vi "think_and_act_with_mark_253.vi"(8 "error in (no error)":errorcluster, 9 "antState":T1, 10 "pieceOfWorld":T4[][](array[typedef]), 11 "Igor in":refnum<class "Igor.lvclass">) -> (0 "error out":errorcluster, 2 "action":T2, 3 "Igor out":refnum<class "Igor.lvclass">)   [LabVIEW 2015]
doc: "Ant thinks and chooses action\nCreated by Artem Shevelev\nshevelev.pro\nartem@shevelev.pro\nLabVIEW Portal: https://labviewportal.org/memberlist.php?mode=viewprofile&u=2340"
uses:
  ant_base/ant_base.lvclass
  ant_base/actionType_enum.ctl
  ant_base/action_cluster.ctl
  actors/world/typedefs/markValue.ctl
  actors/world/world.lvlib
  Igor.lvclass
  moving/move_forvard.vi
  moving/move_back.vi
  actors/world/typedefs/amountOfFood.ctl
  actors/world/typedefs/markValue_cluster.ctl
  actors/world/typedefs/anthillType_enum.ctl
  actors/world/typedefs/worldCell_cluster.ctl
  ant_base/antState_cluster.ctl
  actors/world/typedefs/markVolume.ctl
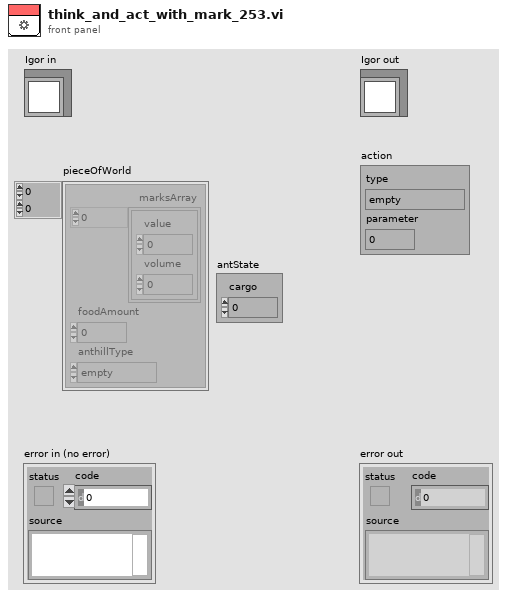
[diagram p1: front panel]
types:
  T1 = typedef "ant_base.lvclass/antState_cluster.ctl" = cluster{"cargo":u8}
  T2 = typedef "ant_base.lvclass/action_cluster.ctl" = cluster{"type":T3, "parameter":dbl}
  T3 = typedef "ant_base.lvclass/actionType_enum.ctl" = enum8{"empty", "move", "take", "put", "mark"}
  T4 = typedef "world.lvlib/worldCell_cluster.ctl" = cluster{"marksArray":T5[], "foodAmount":T8, "anthillType":T9}
  T5 = typedef "world.lvlib/markValue_cluster.ctl" = cluster{"value":T6, "volume":T7}
  T6 = typedef "world.lvlib/markValue.ctl" = u8
  T7 = typedef "world.lvlib/markVolume.ctl" = u16
  T8 = typedef "world.lvlib/amountOfFood.ctl" = i32
  T9 = typedef "world.lvlib/anthillType_enum.ctl" = enum16{"empty", "own", "rival"}
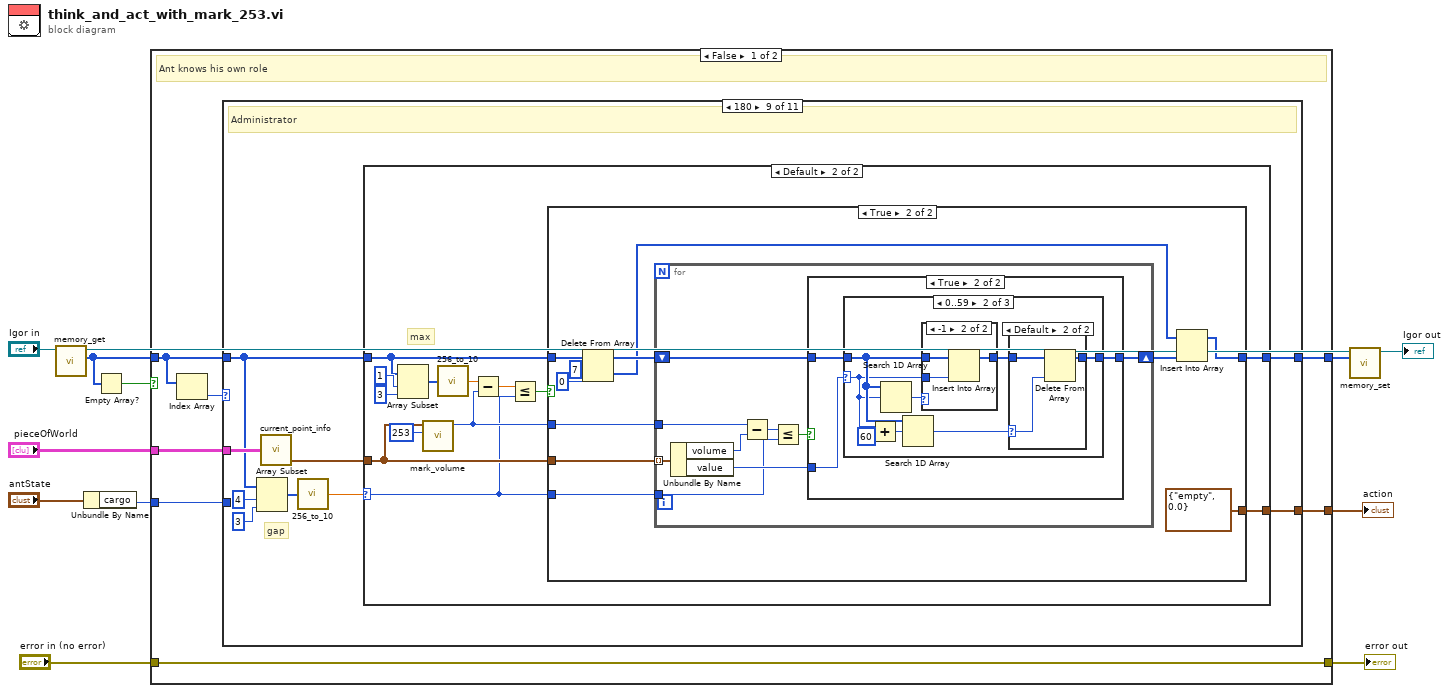
[diagram p0: block diagram]
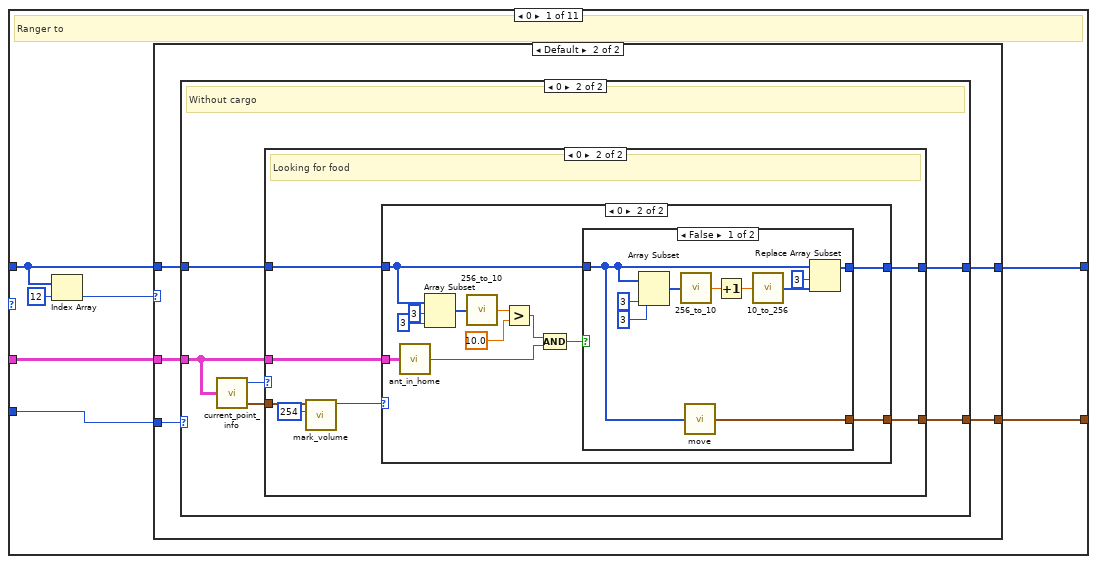
[diagram p2: hidden frame]
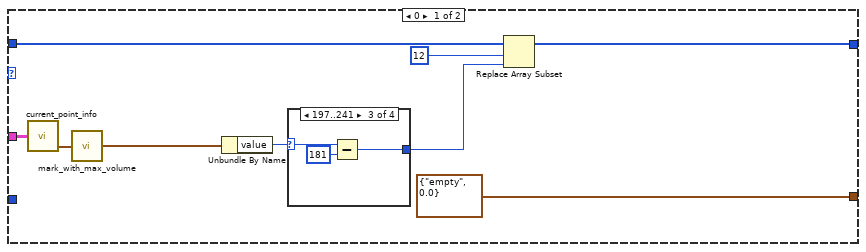
[diagram p3: hidden frame]
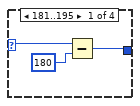
[diagram p4: hidden frame]
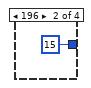
[diagram p5: hidden frame]
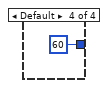
[diagram p6: hidden frame]
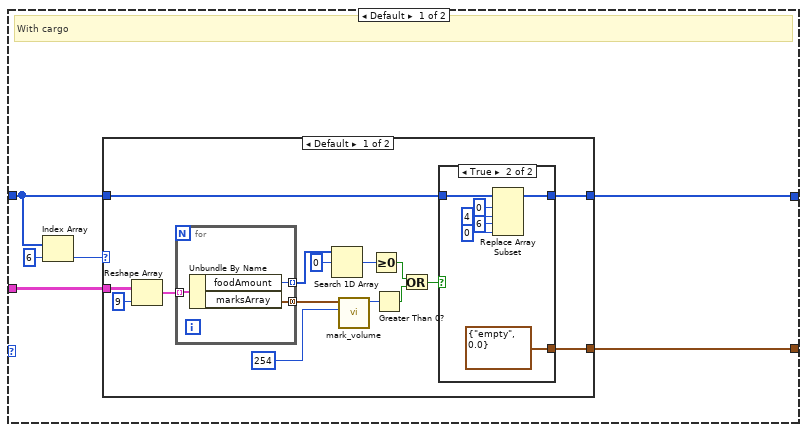
[diagram p7: hidden frame]
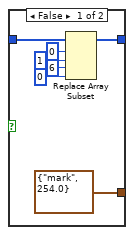
[diagram p8: hidden frame]
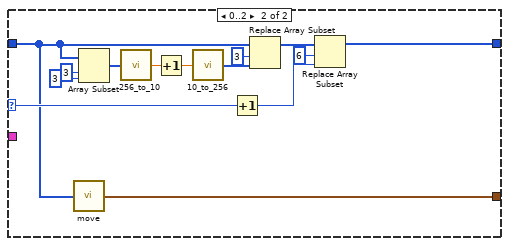
[diagram p9: hidden frame]
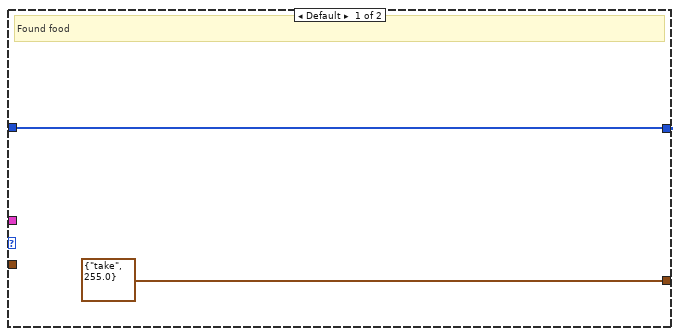
[diagram p10: hidden frame]
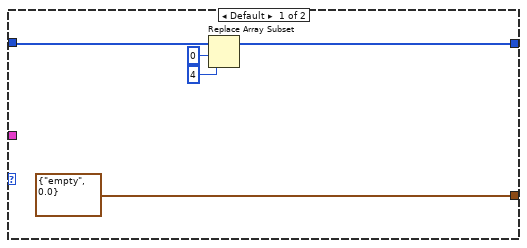
[diagram p11: hidden frame]
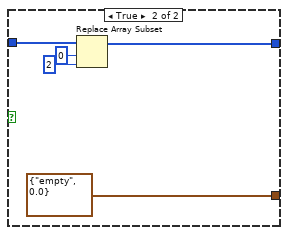
[diagram p12: hidden frame]
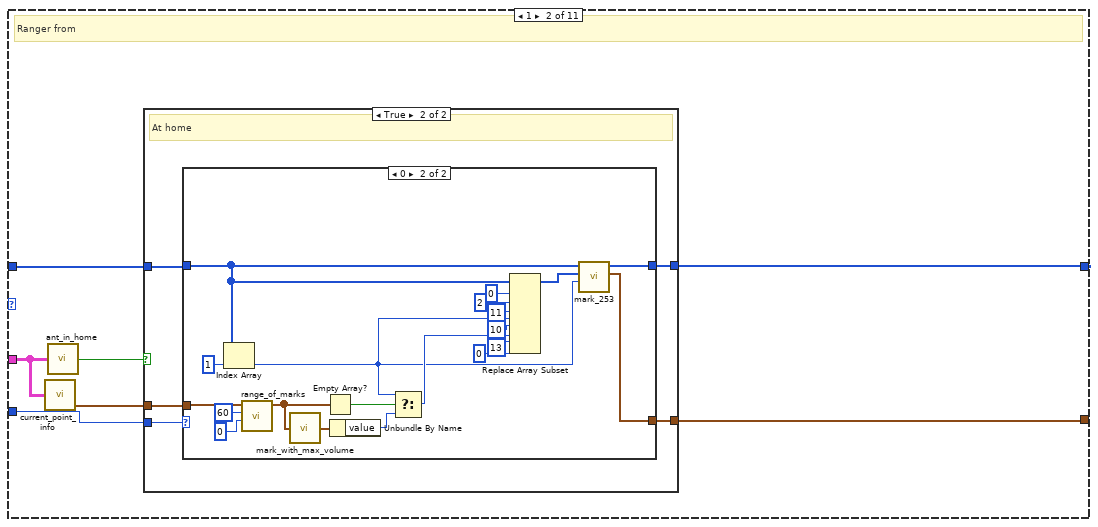
[diagram p13: hidden frame]
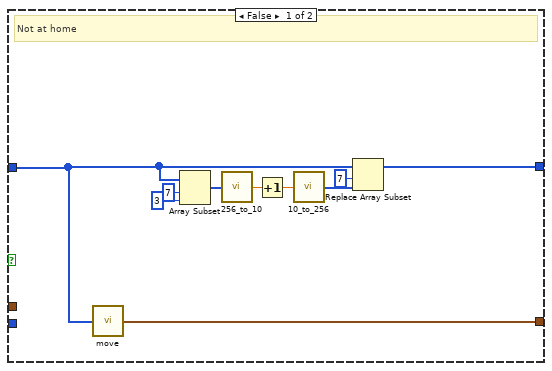
[diagram p14: hidden frame]
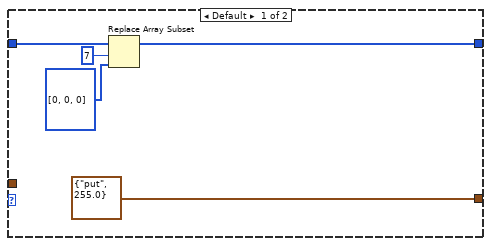
[diagram p15: hidden frame]
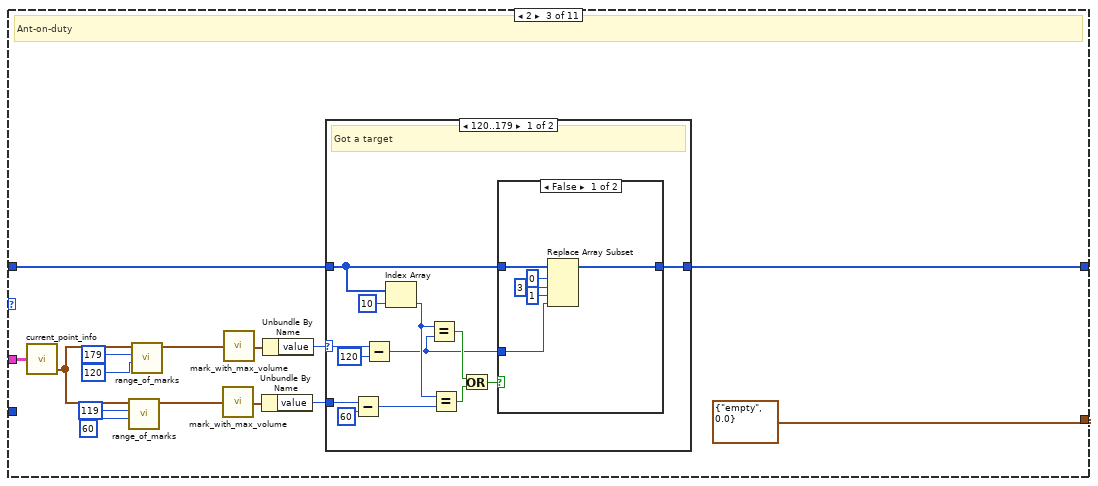
[diagram p16: hidden frame]
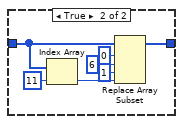
[diagram p17: hidden frame]
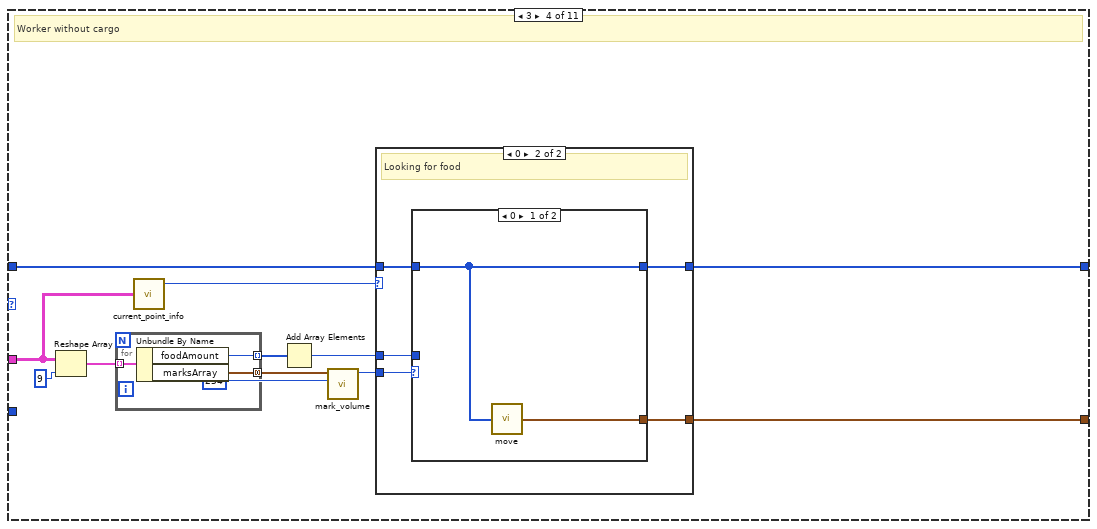
[diagram p19: hidden frame]
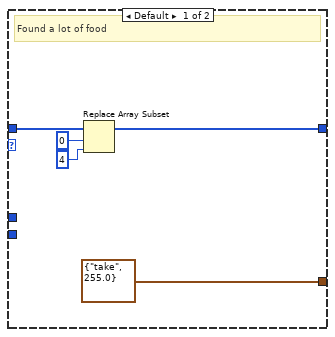
[diagram p20: hidden frame]
diagram:
  n1 = call "memory_get.vi"("ant_base in"="Igor in") -> ("memory"=w2:u8[], "ant_base out"=w7:refnum<class "Igor.lvclass">)  [unwired: 8 in, 1 out]
  n2 = Unbundle By Name("antState") -> ("cargo"=w3:u8)
  n3 = Empty Array?(array=w2) -> (empty?=w9:bool)
  n4 = case shown="False" w9 {
    tunnel: [w19 w757] -> w4
    tunnel: [w17 w756] -> w12
    tunnel: "error in (no error)" -> [w19 w757]
    tunnel: w2 -> [w16 w753]
    tunnel: "pieceOfWorld" -> [w15 w752]
    tunnel: [w14 w754] -> w6
    tunnel: w3 -> [w13 _]
    frame False {
      # "Ant knows his own role"
      n5 = Index Array(array=w16) -> (element=w18:u8)  [unwired: 1 in]
      n6 = case shown="180" w18 {
        tunnel: [w26 w154 T2 {"type"=enum."empty", "parameter"=0.0} ("action") w247 w282 w315 w445 w497 w560 w680 T2 {"type"=enum."empty", "parameter"=0.0} ("action")] -> w17
        tunnel: w16 -> [w22 w148 w207 w248 w281 w314 w448 w498 w556 w676 w749]
        tunnel: w15 -> [w23 w150 w206 w238 w279 w311 w444 w494 w558 w678 _]
        tunnel: [w25 w153 w208 w245 w280 w316 w446 w496 w559 w679 w749] -> w14
        tunnel: w13 -> [w24 w152 _ _ _ _ w449 _ _ _ _]
        frame 0 {
          # "Ranger to"
          n7 = Index Array(array=w22, index=12) -> (element=w20:u8)
          n8 = case shown="Default" w20 {
            tunnel: [T2 {"type"=enum."empty", "parameter"=0.0} ("action") w48] -> w26
            tunnel: w22 -> [w31 w47]
            tunnel: [w30 w46] -> w25
            tunnel: w24 -> [_ w45]
            tunnel: w23 -> [w34 w44]
            frame 0 {
              n9 = call "current_point_info.vi"("pieceOfWorld"=w34) -> ("marksArray"=w33:T5[])  [unwired: 2 out]
              n10 = call "mark_with_max_volume.vi"("marksArray"=w33) -> ("markValue"=w32:T5)
              n11 = Unbundle By Name(w32) -> ("value"=w28:T6)
              n12 = case shown="197..241" w28 {
                selector: w28 -> [w38 _ w42 _]
                tunnel: [w36 15 w40 60 ("value")] -> w27
                frame 181..195 {
                  n13 = Subtract(x=w38, y=180 ("index")) -> (x-y=w36:i32)
                }
                frame 196 {
                }
                frame 197..241 {
                  n14 = Subtract(x=w42, y=T6 181) -> (x-y=w40:T6)
                }
                frame Default {
                }
              }
              n15 = Replace Array Subset(array=w31, new element=w27, index=12) -> (w30:u8[])
            }
            frame Default {
              n16 = case shown="0" w45 {
                tunnel: [w53 w106] -> w48
                tunnel: w47 -> [w52 w105]
                tunnel: [w54 w104] -> w46
                tunnel: w44 -> [w49 w103]
                frame Default {
                  # "With cargo"
                  n17 = Index Array(array=w52, index=6) -> (element=w50:u8)
                  n18 = case shown="Default" w50 {
                    selector: w50 -> [_ w98]
                    tunnel: [w67 w100] -> w54
                    tunnel: w52 -> [w68 w88]
                    tunnel: [w69 w87] -> w53
                    tunnel: w49 -> [w66 _]
                    frame Default {
                      n19 = Reshape Array(w66, 9 ("dimension size")) -> (w65:T4[])
                      n20 = for {
                        tunnel: w65 -> [w86] mode=indexing
                        tunnel: [w85] -> w63 mode=concatenating
                        tunnel: [w84] -> w61 mode=indexing
                        n21 = Unbundle By Name(w86) -> ("foodAmount"=w84:T8, "marksArray"=w85:T5[])
                      }
                      n22 = Search 1D Array(1D array=w61, element=T8 0) -> (index of element=w59:i32)  [unwired: 1 in]
                      n23 = call "mark_volume.vi"("element"=T6 254, "marksArray"=w63) -> ("volume"=w58:T7)  [unwired: 9 in]
                      n24 = Greater Or Equal To 0?(x=w59) -> (x >= 0?=w56:bool)
                      n25 = Greater Than 0?(x=w58) -> (x > 0?=w57:bool)
                      n26 = Or(x=w56, y=w57) -> (x .or. y?=w55:bool)
                      n27 = case shown="True" w55 {
                        tunnel: [T2 {"type"=enum."mark", "parameter"=254.0} ("action") T2 {"type"=enum."empty", "parameter"=0.0} ("action")] -> w69
                        tunnel: w68 -> [w74 w81]
                        tunnel: [w73 w80] -> w67
                        frame False {
                          n28 = Replace Array Subset(array=w74, new element #1=u8 1 ("new element/subarray"), index #1=0 ("index"), new element #2=u8 0 ("new element/subarray"), index #2=6 ("index")) -> (w73:u8[])
                        }
                        frame True {
                          n29 = Replace Array Subset(array=w81, new element #1=u8 4 ("new element/subarray"), index #1=0 ("index"), new element #2=u8 0 ("new element/subarray"), index #2=6 ("index")) -> (w80:u8[])
                        }
                      }
                    }
                    frame 0..2 {
                      n30 = call-poly "move.vi"("Ant's memory"=w88) -> ("action"=w87:T2)
                      n31 = Array Subset(array=w88, index=3, length=3) -> (w93:u8[])
                      n32 = call "256_to_10.vi"("Array"=w93) -> ("Numeric"=w92:dbl)
                      n33 = Increment(x=w92) -> (x+1=w91:dbl)
                      n34 = call "10_to_256.vi"("Decimal"=w91) -> ("256"=w90:u8[])
                      n35 = Increment(x=w98) -> (x+1=w97:u8)
                      n36 = Replace Array Subset(array=w88, new element=w90, index=3) -> (w89:u8[])
                      n37 = Replace Array Subset(array=w89, new element=w97, index=6) -> (w100:u8[])
                    }
                  }
                }
                frame 0 {
                  # "Without cargo"
                  n38 = call "current_point_info.vi"("pieceOfWorld"=w103) -> ("foodAmount"=w102:T8, "marksArray"=w101:T5[])  [unwired: 1 out]
                  n39 = case shown="0" w102 {
                    tunnel: [T2 {"type"=enum."take", "parameter"=255.0} ("action") w115] -> w106
                    tunnel: w105 -> [w107 w113]
                    tunnel: [w107 w114] -> w104
                    tunnel: w103 -> [_ w112]
                    tunnel: w101 -> [_ w111]
                    frame Default {
                      # "Found food"
                    }
                    frame 0 {
                      # "Looking for food"
                      n40 = call "mark_volume.vi"("element"=T6 254, "marksArray"=w111) -> ("volume"=w109:T7)  [unwired: 9 in]
                      n41 = case shown="0" w109 {
                        tunnel: [T2 {"type"=enum."empty", "parameter"=0.0} ("action") w132] -> w115
                        tunnel: [w118 w131] -> w114
                        tunnel: w113 -> [w119 w127]
                        tunnel: w112 -> [_ w122]
                        frame Default {
                          n42 = Replace Array Subset(array=w119, new element=u8 4 ("new element/subarray"), index=0) -> (w118:u8[])
                        }
                        frame 0 {
                          n43 = call "ant_in_home.vi"("pieceOfWorld"=w122) -> ("x .and. y?"=w121:bool)
                          n44 = Array Subset(array=w127, index=3, length=3) -> (w128:u8[])
                          n45 = call "256_to_10.vi"("Array"=w128) -> ("Numeric"=w126:dbl)
                          n46 = Greater?(x=w126, y=10.0) -> (0:w124:bool)
                          n47 = Compound Arithmetic op=AND(w124, w121) -> (w123:bool)
                          n48 = case shown="False" w123 {
                            tunnel: [w133 T2 {"type"=enum."empty", "parameter"=0.0} ("action")] -> w132
                            tunnel: [w135 w146] -> w131
                            tunnel: w127 -> [w134 w147]
                            frame False {
                              n49 = Array Subset(array=w134, index=3, length=3) -> (w139:u8[])
                              n50 = call "256_to_10.vi"("Array"=w139) -> ("Numeric"=w138:dbl)
                              n51 = call-poly "move.vi"("Ant's memory"=w134) -> ("action"=w133:T2)
                              n52 = Increment(x=w138) -> (x+1=w137:dbl)
                              n53 = call "10_to_256.vi"("Decimal"=w137) -> ("256"=w136:u8[])
                              n54 = Replace Array Subset(array=w134, new element=w136, index=3) -> (w135:u8[])
                            }
                            frame True {
                              n55 = Replace Array Subset(array=w147, new element=u8 2 ("new element/subarray"), index=0) -> (w146:u8[])
                            }
                          }
                        }
                      }
                    }
                  }
                }
              }
            }
          }
        }
        frame 1 {
          # "Ranger from"
          n56 = call "current_point_info.vi"("pieceOfWorld"=w150) -> ("marksArray"=w149:T5[])  [unwired: 2 out]
          n57 = call "ant_in_home.vi"("pieceOfWorld"=w150) -> ("x .and. y?"=w151:bool)
          n58 = case shown="True" w151 {
            tunnel: [w164 w169] -> w154
            tunnel: w149 -> [_ w167]
            tunnel: w148 -> [w156 w166]
            tunnel: [w155 w168] -> w153
            tunnel: w152 -> [_ w165]
            frame False {
              # "Not at home"
              n59 = call-poly "move.vi"("Ant's memory"=w156) -> ("action"=w164:T2)
              n60 = Array Subset(array=w156, index=7, length=3) -> (w160:u8[])
              n61 = call "256_to_10.vi"("Array"=w160) -> ("Numeric"=w159:dbl)
              n62 = Increment(x=w159) -> (x+1=w158:dbl)
              n63 = call "10_to_256.vi"("Decimal"=w158) -> ("256"=w157:u8[])
              n64 = Replace Array Subset(array=w156, new element=w157, index=7) -> (w155:u8[])
            }
            frame True {
              # "At home"
              n65 = case shown="0" w165 {
                tunnel: [T2 {"type"=enum."put", "parameter"=255.0} ("action") w176] -> w169
                tunnel: w166 -> [w173 w179]
                tunnel: [w172 w177] -> w168
                tunnel: w167 -> [_ w194]
                frame Default {
                  n66 = Replace Array Subset(array=w173, new element=i32[] [0, 0, 0], index=7) -> (w172:u8[])
                }
                frame 0 {
                  n67 = Index Array(array=w179, index=1) -> (element=w175:u8)
                  n68 = call "range_of_marks.vi"("lower limit"=T6 0, "upper limit"=T6 60, "marksArray"=w194) -> ("Array"=w182:T5[])  [unwired: 8 in]
                  n69 = call "mark_with_max_volume.vi"("marksArray"=w182) -> ("markValue"=w188:T5)
                  n70 = Empty Array?(array=w182) -> (empty?=w187:bool)
                  n71 = Unbundle By Name(w188) -> ("value"=w186:T6)
                  n72 = Select(t=w175, s=w187, f=w186) -> (s? t:f=w185:T6)
                  n73 = Replace Array Subset(array=w179, new element #1=u8 2 ("new element/subarray"), index #1=0 ("index"), new element #2=w175, index #2=11 ("index"), new element #3=w185, index #3=10 ("index"), new element #4=u8 0 ("new element/subarray"), index #4=13 ("index")) -> (w178:u8[])
                  n74 = call "mark_253.vi"("mark value"=w175, "memory in 2"=w178, "memory in"=w179) -> ("action"=w176:T2, "memory out"=w177:u8[])  [unwired: 7 in]
                }
              }
            }
          }
        }
        frame 2 {
          # "Ant-on-duty"
          n75 = call "current_point_info.vi"("pieceOfWorld"=w206) -> ("marksArray"=w198:T5[])  [unwired: 2 out]
          n76 = call "range_of_marks.vi"("lower limit"=T6 60, "upper limit"=T6 119, "marksArray"=w198) -> ("Array"=w197:T5[])  [unwired: 8 in]
          n77 = call "range_of_marks.vi"("lower limit"=T6 120, "upper limit"=T6 179, "marksArray"=w198) -> ("Array"=w202:T5[])  [unwired: 8 in]
          n78 = call "mark_with_max_volume.vi"("marksArray"=w197) -> ("markValue"=w199:T5)
          n79 = call "mark_with_max_volume.vi"("marksArray"=w202) -> ("markValue"=w203:T5)
          n80 = Unbundle By Name(w199) -> ("value"=w195:T6)
          n81 = Unbundle By Name(w203) -> ("value"=w196:T6)
          n82 = case shown="120..179" w196 {
            selector: w196 -> [w215 _]
            tunnel: w207 -> [w221 w236]
            tunnel: [w222 w236] -> w208
            tunnel: w195 -> [w211 _]
            frame 120..179 {
              # "Got a target"
              n83 = Subtract(x=w211, y=T6 60) -> (x-y=w210:T6)
              n84 = Subtract(x=w215, y=T6 120) -> (x-y=w213:T6)
              n85 = Index Array(array=w221, index=10) -> (element=w219:u8)
              n86 = Equal?(x=w219, y=w213) -> (x = y?=w218:bool)
              n87 = Equal?(x=w219, y=w210) -> (x = y?=w216:bool)
              n88 = Or(x=w218, y=w216) -> (x .or. y?=w217:bool)
              n89 = case shown="False" w217 {
                tunnel: w213 -> [w223 _]
                tunnel: w221 -> [w228 w230]
                tunnel: [w224 w232] -> w222
                frame False {
                  n90 = Replace Array Subset(array=w228, new element #1=u8 3 ("new element/subarray"), index #1=0 ("index"), new element #2=w223, index #2=1 ("index")) -> (w224:u8[])
                }
                frame True {
                  n91 = Index Array(array=w230, index=11) -> (element=w229:u8)
                  n92 = Replace Array Subset(array=w230, new element #1=u8 6 ("new element/subarray"), index #1=0 ("index"), new element #2=w229, index #2=1 ("index")) -> (w232:u8[])
                }
              }
            }
            frame Default {
              # "Expecting a target"
            }
          }
        }
        frame 3 {
          # "Worker without cargo"
          n93 = Reshape Array(w238, 9 ("dimension size")) -> (w243:T4[])
          n94 = for {
            tunnel: w243 -> [w251] mode=indexing
            tunnel: [w250] -> w240 mode=concatenating
            tunnel: [w249] -> w242 mode=indexing
            n95 = Unbundle By Name(w251) -> ("foodAmount"=w249:T8, "marksArray"=w250:T5[])
          }
          n96 = call "current_point_info.vi"("pieceOfWorld"=w238) -> ("foodAmount"=w237:T8)  [unwired: 2 out]
          n97 = Add Array Elements(numeric array=w242) -> (sum=w241:T8)
          n98 = call "mark_volume.vi"("element"=T6 254, "marksArray"=w240) -> ("volume"=w239:T7)  [unwired: 9 in]
          n99 = case shown="0" w237 {
            tunnel: [T2 {"type"=enum."take", "parameter"=255.0} ("action") w261] -> w247
            tunnel: w248 -> [w255 w259]
            tunnel: w239 -> [_ w260]
            tunnel: [w252 w258] -> w245
            tunnel: w241 -> [_ w257]
            frame Default {
              # "Found a lot of food"
              n100 = Replace Array Subset(array=w255, new element=4 ("index"), index=0) -> (w252:u8[])
            }
            frame 0 {
              # "Looking for food"
              n101 = case shown="0" w260 {
                tunnel: [w262 T2 {"type"=enum."empty", "parameter"=0.0} ("action")] -> w261
                tunnel: w259 -> [w263 w270]
                tunnel: [w263 w269] -> w258
                tunnel: w257 -> [_ w268]
                frame 0 {
                  n102 = call-poly "move.vi"("Ant's memory"=w263) -> ("action"=w262:T2)
                }
                frame Default {
                  n103 = Index Array(array=w270, index=1) -> (element=w272:u8)
                  n104 = Equal To 0?(x=w268) -> (x = 0?=w267:bool)
                  n105 = Add(x=w272, y=u8 60) -> (x+y=w266:u8)
                  n106 = Select(t=w266, s=w267, f=u8 0) -> (s? t:f=w264:u8)
                  n107 = Replace Array Subset(array=w270, new element #1=u8 4 ("new element/subarray"), index #1=0 ("index"), new element #2=w264, index #2=2 ("index")) -> (w269:u8[])
                }
              }
            }
          }
        }
        frame 4 {
          # "Worker with cargo"
          n108 = call "ant_in_home.vi"("pieceOfWorld"=w279) -> ("x .and. y?"=w278:bool)
          n109 = case shown="True" w278 {
            tunnel: [w283 w288] -> w282
            tunnel: w281 -> [w284 w285]
            tunnel: [w284 w286] -> w280
            frame False {
              # "Not at home"
              n110 = call-poly "move.vi"("Ant's memory"=w284) -> ("action"=w283:T2)
            }
            frame True {
              # "At home"
              n111 = Index Array(array=w285, index=2) -> (element=w287:u8)
              n112 = case shown="60..119" w287 {
                selector: w287 -> [w290 _]
                tunnel: [w291 T2 {"type"=enum."put", "parameter"=255.0} ("action")] -> w288
                tunnel: [w293 w301] -> w286
                tunnel: w285 -> [w294 w302]
                frame 60..119 {
                  n113 = Replace Array Subset(array=w294, new element #1=u8 2 ("y"), index #1=0 ("index"), new element #2=u8 0 ("new element/subarray"), index #2=2 ("index"), new element #3=u8 0 ("new element/subarray"), index #3=13 ("index")) -> (w292:u8[])
                  n114 = call "mark_253.vi"("mark value"=w290, "memory in 2"=w292, "memory in"=w294) -> ("action"=w291:T2, "memory out"=w293:u8[])  [unwired: 7 in]
                }
                frame Default {
                  n115 = Replace Array Subset(array=w302, new element #1=u8 2 ("y"), index #1=0 ("index"), new element #2=u8 0 ("new element/subarray"), index #2=2 ("index")) -> (w301:u8[])
                }
              }
            }
          }
        }
        frame 55 {
          n116 = call "current_point_info.vi"("pieceOfWorld"=w311) -> ("anthillType"=w317:T9)  [unwired: 2 out]
          n117 = Reshape Array(w311, 9 ("dimension size")) -> (w309:T4[])
          n118 = Index Array(array=w314, index=4) -> (element=w312:u8)
          n119 = for {
            tunnel: w309 -> [w319] mode=indexing
            tunnel: [w318] -> w308 mode=concatenating
            n120 = Unbundle By Name(w319) -> ("marksArray"=w318:T5[])
          }
          n121 = case shown="2" w312 {
            tunnel: w317 -> [w323 _ _]
            tunnel: w314 -> [w322 w377 w406]
            tunnel: [w321 w376 w405] -> w316
            tunnel: [w320 w375 w404] -> w315
            tunnel: w308 -> [_ _ w403]
            frame 0, Default {
              n122 = case shown="Default" w323 {
                tunnel: w322 -> [w328 w340]
                tunnel: [w335 w339] -> w321
                tunnel: [w333 w338] -> w320
                frame "own" {
                  n123 = Index Array(array=w328, index=1) -> (element=w330:u8)
                  n124 = Index Array(array=w328, index=2) -> (element=w326:u8)
                  n125 = Increment(x=w326) -> (x+1=w324:u8)
                  n126 = Multiply(x=w330, y=1.5707963267948966) -> (x*y=w329:dbl)
                  n127 = Replace Array Subset(array=w328, new element=w324, index=2) -> (w335:u8[])
                  n128 = Bundle By Name(cluster=T2 {"type"=enum."move", "parameter"=0.0} ("action"), "parameter"=w329) -> (w333:T2)
                }
                frame Default {
                  n129 = Index Array(array=w340, index #1=3 ("index"), index #2=2 ("index")) -> (element #1=w337:u8, element #2=w336:u8)
                  n130 = Greater Or Equal?(x=w337, y=w336) -> (x >= y?=w341:bool)
                  n131 = case shown="False" w341 {
                    tunnel: w340 -> [w347 w361]
                    tunnel: [w354 w367] -> w339
                    tunnel: [w344 T2 {"type"=enum."empty", "parameter"=0.0} ("action")] -> w338
                    tunnel: w337 -> [w352 _]
                    frame False {
                      n132 = Increment(x=w352) -> (x+1=w351:u8)
                      n133 = Index Array(array=w347, index=1) -> (element=w348:u8)
                      n134 = Multiply(x=w348, y=1.5707963267948966) -> (x*y=w346:dbl)
                      n135 = Replace Array Subset(array=w347, new element=w351, index=3) -> (w354:u8[])
                      n136 = Bundle By Name(cluster=T2 {"type"=enum."move", "parameter"=0.0} ("action"), "parameter"=w346) -> (w344:T2)
                    }
                    frame True {
                      n137 = Index Array(array=w361, index=1) -> (element=w359:u8)
                      n138 = Increment(x=w359) -> (x+1=w358:u8)
                      n139 = Quotient & Remainder(x=w358, y=u8 4) -> (x-y*floor(x/y)=w356:u8)  [unwired: 1 out]
                      n140 = Replace Array Subset(array=w361, new element #1=u8 0 ("new element/subarray"), index #1=3 ("index"), new element #2=u8 1 ("new element/subarray"), index #2=4 ("index"), new element #3=w356, index #3=1 ("index")) -> (w367:u8[])
                    }
                  }
                }
              }
            }
            frame 1 {
              n141 = Index Array(array=w377, index #1=3 ("index"), index #2=2 ("index")) -> (element #1=w371:u8, element #2=w369:u8)
              n142 = Multiply(x=w369, y=u8 2) -> (x*y=w368:u8)
              n143 = Greater Or Equal?(x=w371, y=w368) -> (x >= y?=w372:bool)
              n144 = case shown="False" w372 {
                tunnel: w377 -> [w382 w395]
                tunnel: [w378 w401] -> w376
                tunnel: [w379 T2 {"type"=enum."empty", "parameter"=0.0} ("action")] -> w375
                tunnel: w371 -> [w387 _]
                frame False {
                  n145 = Increment(x=w387) -> (x+1=w386:u8)
                  n146 = Replace Array Subset(array=w382, new element=w386, index=3) -> (w378:u8[])
                  n147 = Index Array(array=w378, index=1) -> (element=w383:u8)
                  n148 = Multiply(x=w383, y=1.5707963267948966) -> (x*y=w381:dbl)
                  n149 = Bundle By Name(cluster=T2 {"type"=enum."move", "parameter"=0.0} ("action"), "parameter"=w381) -> (w379:T2)
                }
                frame True {
                  n150 = Index Array(array=w395, index=1) -> (element=w393:u8)
                  n151 = Increment(x=w393) -> (x+1=w392:u8)
                  n152 = Quotient & Remainder(x=w392, y=u8 4) -> (x-y*floor(x/y)=w390:u8)  [unwired: 1 out]
                  n153 = Replace Array Subset(array=w395, new element #1=u8 0 ("new element/subarray"), index #1=3 ("index"), new element #2=u8 2 ("new element/subarray"), index #2=4 ("index"), new element #3=w390, index #3=1 ("index")) -> (w401:u8[])
                }
              }
            }
            frame 2 {
              n154 = Empty Array?(array=w403) -> (empty?=w402:bool)
              n155 = case shown="False" w402 {
                tunnel: w406 -> [w416 w441]
                tunnel: [w415 w441] -> w405
                tunnel: [w414 T2 {"type"=enum."mark", "parameter"=23.0} ("action")] -> w404
                frame False {
                  n156 = Index Array(array=w416, index #1=3 ("index"), index #2=2 ("index")) -> (element #1=w410:u8, element #2=w409:u8)
                  n157 = Multiply(x=w409, y=u8 4) -> (x*y=w407:u8)
                  n158 = Greater Or Equal?(x=w410, y=w407) -> (x >= y?=w411:bool)
                  n159 = case shown="True" w411 {
                    tunnel: w416 -> [w421 w434]
                    tunnel: [w417 w440] -> w415
                    tunnel: [w418 T2 {"type"=enum."empty", "parameter"=0.0} ("action")] -> w414
                    tunnel: w410 -> [w426 _]
                    frame False {
                      n160 = Increment(x=w426) -> (x+1=w425:u8)
                      n161 = Replace Array Subset(array=w421, new element=w425, index=3) -> (w417:u8[])
                      n162 = Index Array(array=w417, index=1) -> (element=w422:u8)
                      n163 = Multiply(x=w422, y=1.5707963267948966) -> (x*y=w420:dbl)
                      n164 = Bundle By Name(cluster=T2 {"type"=enum."move", "parameter"=0.0} ("action"), "parameter"=w420) -> (w418:T2)
                    }
                    frame True {
                      n165 = Index Array(array=w434, index=1) -> (element=w432:u8)
                      n166 = Increment(x=w432) -> (x+1=w431:u8)
                      n167 = Quotient & Remainder(x=w431, y=u8 4) -> (x-y*floor(x/y)=w429:u8)  [unwired: 1 out]
                      n168 = Replace Array Subset(array=w434, new element #1=u8 0 ("new element/subarray"), index #1=3 ("index"), new element #2=u8 2 ("new element/subarray"), index #2=4 ("index"), new element #3=w429, index #3=1 ("index")) -> (w440:u8[])
                    }
                  }
                }
                frame True {
                }
              }
            }
          }
        }
        frame 6 {
          # "Expirienced ranger to foodHeap"
          n169 = Array Subset(array=w448, index=3, length=3 ("index")) -> (w453:u8[])
          n170 = Array Subset(array=w448, index=7, length=3) -> (w455:u8[])
          n171 = call "current_point_info.vi"("pieceOfWorld"=w444) -> ("foodAmount"=w443:T8)  [unwired: 2 out]
          n172 = call "256_to_10.vi"("Array"=w455) -> ("Numeric"=w452:dbl)
          n173 = call "256_to_10.vi"("Array"=w453) -> ("Numeric"=w450:dbl)
          n174 = Greater Or Equal?(x=w452, y=w450) -> (x >= y?=w447:bool)
          n175 = case shown="False" w447 {
            tunnel: w449 -> [w462 w481]
            tunnel: w443 -> [w463 _]
            tunnel: w448 -> [w465 w487]
            tunnel: [w458 T2 {"type"=enum."mark", "parameter"=254.0} ("action")] -> w445
            tunnel: [w464 w488] -> w446
            frame False {
              n176 = Greater Than 0?(x=w462) -> (x > 0?=w460:bool)
              n177 = Greater Than 0?(x=w463) -> (x > 0?=w461:bool)
              n178 = Implies(1:w460, 2:w461) -> (0:w459:bool)
              n179 = case shown="True" w459 {
                tunnel: [w466 w477] -> w464
                tunnel: w465 -> [w466 w469]
                tunnel: [T2 {"type"=enum."take", "parameter"=255.0} ("action") w468] -> w458
                frame False {
                  # "Found food"
                }
                frame True {
                  # "No food in cell"
                  n180 = Array Subset(array=w469, index=7, length=3) -> (w473:u8[])
                  n181 = call-poly "move.vi"("Ant's memory"=w469) -> ("action"=w468:T2)
                  n182 = call "256_to_10.vi"("Array"=w473) -> ("Numeric"=w472:dbl)
                  n183 = Increment(x=w472) -> (x+1=w471:dbl)
                  n184 = call "10_to_256.vi"("Decimal"=w471) -> ("256"=w470:u8[])
                  n185 = Replace Array Subset(array=w469, new element=w470, index=7) -> (w477:u8[])
                }
              }
            }
            frame True {
              n186 = Less?(x=w481, y=u8 255) -> (x < y?=w479:bool)
              n187 = Index Array(array=w487, index=1) -> (element=w486:u8)
              n188 = Add(x=w486, y=u8 60) -> (x+y=w484:u8)
              n189 = Select(t=w484, s=w479, f=u8 0) -> (s? t:f=w482:u8)
              n190 = Replace Array Subset(array=w487, new element #1=u8 7 ("new element/subarray"), index #1=0 ("index"), new element #2=w482, index #2=2 ("index")) -> (w488:u8[])
            }
          }
        }
        frame 7 {
          # "Expirienced ranger from foodHeap"
          n191 = call "current_point_info.vi"("pieceOfWorld"=w494) -> ("marksArray"=w493:T5[])  [unwired: 2 out]
          n192 = call "ant_in_home.vi"("pieceOfWorld"=w494) -> ("x .and. y?"=w495:bool)
          n193 = case shown="False" w495 {
            tunnel: [w499 w509] -> w497
            tunnel: w498 -> [w500 w506]
            tunnel: [w500 w508] -> w496
            tunnel: w493 -> [_ w507]
            frame False {
              # "Not at home"
              n194 = call-poly "move.vi"("Ant's memory"=w500) -> ("action"=w499:T2)
            }
            frame True {
              # "At home"
              n195 = Index Array(array=w506, index=1) -> (element=w501:u8)
              n196 = Add(x=w501, y=u8 60) -> (x+y=w503:u8)
              n197 = call "mark_volume.vi"("element"=w503, "marksArray"=w507) -> ("volume"=w502:T7)  [unwired: 9 in]
              n198 = case shown="0" w502 {
                tunnel: [T2 {"type"=enum."put", "parameter"=255.0} ("action") w521] -> w509
                tunnel: w506 -> [w513 w519]
                tunnel: [w516 w520] -> w508
                tunnel: w501 -> [w515 _]
                frame Default {
                  w510 = u8 0 ("y")
                  n199 = Index Array(array=w513, index=12) -> (element=w511:u8)
                  n200 = Build Array(w510, w515, w510, w510, w510, w510, w510, w510, w510, w510, w510, w510, w511, w510) -> (w516:u8[])
                }
                frame 0 {
                  n201 = Index Array(array=w519, index=2) -> (element=w517:u8)
                  n202 = case shown="0" w517 {
                    selector: w517 -> [_ w535]
                    tunnel: w519 -> [w532 w537]
                    tunnel: [T2 {"type"=enum."put", "parameter"=255.0} ("action") w536] -> w521
                    tunnel: [w530 w538] -> w520
                    frame 0 {
                      n203 = Replace Array Subset(array=w532, new element #1=u8 6 ("new element/subarray"), index #1=0 ("index"), new element #2=u8 0 ("new element/subarray"), index #2=2 ("index"), new element #3=u8 0 ("new element/subarray"), index #3=7 ("index"), new element #4=u8 0 ("new element/subarray"), index #4=8 ("index"), new element #5=u8 0 ("new element/subarray"), index #5=9 ("index")) -> (w530:u8[])
                    }
                    frame Default {
                      n204 = Replace Array Subset(array=w537, new element #1=u8 7 ("new element/subarray"), index #1=0 ("index"), new element #2=u8 0 ("new element/subarray"), index #2=2 ("index"), new element #3=u8 0 ("new element/subarray"), index #3=7 ("index"), new element #4=u8 0 ("new element/subarray"), index #4=8 ("index"), new element #5=u8 0 ("new element/subarray"), index #5=9 ("index"), new element #6=u8 0 ("new element/subarray"), index #6=13 ("index")) -> (w539:u8[])
                      n205 = call "mark_253.vi"("mark value"=w535, "memory in 2"=w539, "memory in"=w537) -> ("action"=w536:T2, "memory out"=w538:u8[])  [unwired: 7 in]
                    }
                  }
                }
              }
            }
          }
        }
        frame 180 {
          # "gap"
          # "Administrator"
          n206 = Array Subset(array=w556, index=4, length=3) -> (w553:u8[])
          n207 = call "current_point_info.vi"("pieceOfWorld"=w558) -> ("marksArray"=w557:T5[])  [unwired: 2 out]
          n208 = call "256_to_10.vi"("Array"=w553) -> ("Numeric"=w552:dbl)
          n209 = case shown="Default" w552 {
            selector: w552 -> [_ w578]
            tunnel: [T2 {"type"=enum."empty", "parameter"=0.0} ("action") w590] -> w560
            tunnel: w556 -> [w565 w579]
            tunnel: [w568 w589] -> w559
            tunnel: w557 -> [w570 w588]
            frame 0 {
              n210 = call "mark_with_max_volume.vi"("marksArray"=w570) -> ("markValue"=w569:T5)
              n211 = Unbundle By Name(w569) -> ("volume"=w567:T7)
              n212 = Array Subset(array=w565, index=1, length=3) -> (w562:u8[])
              n213 = call "256_to_10.vi"("Array"=w562) -> ("Numeric"=w561:dbl)
              n214 = Subtract(x=w561, y=w567) -> (x-y=w566:dbl)
              n215 = case shown="Default" w566 {
                selector: w566 -> [_ w573]
                tunnel: w565 -> [w572 w577]
                tunnel: [w572 w574] -> w568
                frame 0 {
                }
                frame Default {
                  n216 = call "10_to_256.vi"("Decimal"=w573) -> ("256"=w575:u8[])
                  n217 = Replace Array Subset(array=w577, new element=w575, index=4) -> (w574:u8[])
                }
              }
            }
            frame Default {
              # "max"
              n218 = Array Subset(array=w579, index=1, length=3) -> (w582:u8[])
              n219 = call "mark_volume.vi"("element"=T6 253, "marksArray"=w588) -> ("volume"=w581:T7)  [unwired: 9 in]
              n220 = call "256_to_10.vi"("Array"=w582) -> ("Numeric"=w580:dbl)
              n221 = Subtract(x=w580, y=w581) -> (x-y=w586:dbl)
              n222 = Less Or Equal?(x=w586, y=w578) -> (x <= y?=w585:bool)
              n223 = case shown="True" w585 {
                tunnel: [w597 T2 {"type"=enum."empty", "parameter"=0.0} ("action")] -> w590
                tunnel: w579 -> [w593 w625]
                tunnel: [w593 w619] -> w589
                tunnel: w588 -> [w595 w629]
                tunnel: w581 -> [_ w627]
                tunnel: w578 -> [_ w626]
                frame False {
                  n224 = Array Subset(array=w593, index=7) -> (w591:u8[])  [unwired: 1 in]
                  n225 = call "mark_volume.vi"("element"=T6 180, "marksArray"=w595) -> ("volume"=w596:T7)  [unwired: 9 in]
                  n226 = case shown="Default" w596 {
                    tunnel: [w600 T2 {"type"=enum."mark", "parameter"=180.0} ("action")] -> w597
                    tunnel: w591 -> [w598 _]
                    tunnel: w595 -> [w599 _]
                    frame Default {
                      n227 = for {
                        tunnel: [w604] -> w600
                        tunnel: w599 -> [w603]
                        tunnel: w598 -> [w601] mode=indexing
                        stop <- w602 stop-if-true
                        n228 = case shown="0..59" w601 {
                          selector: w601 -> [_ w607]
                          tunnel: [T2 {"type"=enum."empty", "parameter"=0.0} ("action") w613] -> w604
                          tunnel: w603 -> [_ w612]
                          tunnel: [FALSE TRUE] -> w602
                          frame Default {
                          }
                          frame 0..59 {
                            n229 = Add(x=w607, y=u8 120) -> (x+y=w610:u8)
                            n230 = call "mark_volume.vi"("element"=w610, "marksArray"=w612) -> ("volume"=w609:T7)  [unwired: 9 in]
                            n231 = case shown="0..1000" w609 {
                              tunnel: [T2 {"type"=enum."empty", "parameter"=0.0} ("action") w617] -> w613
                              tunnel: w610 -> [_ w616]
                              frame Default {
                              }
                              frame 0..1000 {
                                n232 = Bundle By Name(cluster=T2 {"type"=enum."mark", "parameter"=0.0} ("action"), "parameter"=w616) -> (w617:T2)
                              }
                            }
                          }
                        }
                      }
                    }
                    frame 0..1000 {
                    }
                  }
                }
                frame True {
                  n233 = Delete From Array(array=w625, length=7, index=0) -> (deleted portion=w621:u8[], array with subset deleted=w622:u8[])
                  n234 = for {
                    tunnel: w629 -> [w638] mode=indexing
                    shift-right: [w636] -> w620
                    shift-left: w622 -> [w637]
                    tunnel: w627 -> [w631]
                    tunnel: w626 -> [w632]
                    n235 = Unbundle By Name(w638) -> ("volume"=w630:T7, "value"=w635:T6)
                    n236 = Subtract(x=w631, y=w630) -> (x-y=w634:T7)
                    n237 = Less Or Equal?(x=w634, y=w632) -> (x <= y?=w633:bool)
                    n238 = case shown="True" w633 {
                      tunnel: w637 -> [w639 w642]
                      tunnel: [w639 w641] -> w636
                      tunnel: w635 -> [_ w640]
                      frame False {
                      }
                      frame True {
                        n239 = case shown="0..59" w640 {
                          selector: w640 -> [_ w648 w661]
                          tunnel: w642 -> [w643 w649 w663]
                          tunnel: [w643 w646 w662] -> w641
                          frame Default {
                          }
                          frame 0..59 {
                            n240 = Add(x=w648, y=T6 60) -> (x+y=w651:T6)
                            n241 = Search 1D Array(1D array=w649, element=w648) -> (index of element=w644:i32)  [unwired: 1 in]
                            n242 = Search 1D Array(1D array=w649, element=w651) -> (index of element=w645:i32)  [unwired: 1 in]
                            n243 = case shown="-1" w644 {
                              tunnel: w649 -> [w656 w659]
                              tunnel: [w656 w658] -> w647
                              tunnel: w648 -> [_ w657]
                              frame Default {
                              }
                              frame -1 {
                                n244 = Insert Into Array(array=w659, new element=w657) -> (w658:u8[])  [unwired: 1 in]
                              }
                            }
                            n245 = case shown="Default" w645 {
                              selector: w645 -> [_ w653]
                              tunnel: w647 -> [w652 w655]
                              tunnel: [w652 w654] -> w646
                              frame -1 {
                              }
                              frame Default {
                                n246 = Delete From Array(array=w655, index=w653) -> (array with subset deleted=w654:u8[])  [unwired: 1 in, 1 out]
                              }
                            }
                          }
                          frame 60..119 {
                            n247 = Search 1D Array(1D array=w663, element=w661) -> (index of element=w660:i32)  [unwired: 1 in]
                            n248 = case shown="-1" w660 {
                              tunnel: w663 -> [w664 w669]
                              tunnel: [w664 w667] -> w662
                              tunnel: w661 -> [_ w666]
                              frame 0, Default {
                              }
                              frame -1 {
                                n249 = Subtract(x=w666, y=T6 60) -> (x-y=w671:T6)
                                n250 = Insert Into Array(array=w669, new element=w666) -> (w668:u8[])  [unwired: 1 in]
                                n251 = Search 1D Array(1D array=w669, element=w671) -> (index of element=w665:i32)  [unwired: 1 in]
                                n252 = Delete From Array(array=w668, index=w665) -> (array with subset deleted=w667:u8[])  [unwired: 1 in, 1 out]
                              }
                            }
                          }
                        }
                      }
                    }
                  }
                  n253 = Insert Into Array(array=w621, new element=w620) -> (w619:u8[])  [unwired: 1 in]
                }
              }
            }
          }
        }
        frame 181 {
          # "Administrator"
          n254 = call "current_point_info.vi"("pieceOfWorld"=w678) -> ("marksArray"=w677:T5[])  [unwired: 2 out]
          n255 = Array Subset(array=w676, index=1, length=3) -> (w673:u8[])
          n256 = call "256_to_10.vi"("Array"=w673) -> ("Numeric"=w672:dbl)
          n257 = case shown="Default" w672 {
            tunnel: [T2 {"type"=enum."empty", "parameter"=0.0} ("action") w694] -> w680
            tunnel: w676 -> [w684 w692]
            tunnel: [w681 w693] -> w679
            tunnel: w677 -> [w687 w691]
            frame 0 {
              n258 = call "mark_with_max_volume.vi"("marksArray"=w687) -> ("markValue"=w686:T5)
              n259 = Unbundle By Name(w686) -> ("volume"=w685:T7)
              n260 = call "10_to_256.vi"("Decimal"=w685) -> ("256"=w682:u8[])
              n261 = Replace Array Subset(array=w684, new element=w682, index=1) -> (w681:u8[])
            }
            frame Default {
              n262 = for {
                tunnel: w691 -> [w719] mode=indexing
                shift-right: [w717] -> w693
                shift-left: w692 -> [w718]
                n263 = Unbundle By Name(w719) -> ("value"=w716:T6)
                n264 = case shown="0..59" w716 {
                  selector: w716 -> [_ w725 w738]
                  tunnel: w718 -> [w720 w726 w740]
                  tunnel: [w720 w723 w739] -> w717
                  frame Default {
                  }
                  frame 0..59 {
                    n265 = Add(x=w725, y=T6 60) -> (x+y=w728:T6)
                    n266 = Search 1D Array(1D array=w726, element=w725) -> (index of element=w721:i32)  [unwired: 1 in]
                    n267 = Search 1D Array(1D array=w726, element=w728) -> (index of element=w722:i32)  [unwired: 1 in]
                    n268 = case shown="-1" w721 {
                      tunnel: w726 -> [w733 w736]
                      tunnel: [w733 w735] -> w724
                      tunnel: w725 -> [_ w734]
                      frame Default {
                      }
                      frame -1 {
                        n269 = Insert Into Array(array=w736, new element=w734) -> (w735:u8[])  [unwired: 1 in]
                      }
                    }
                    n270 = case shown="Default" w722 {
                      selector: w722 -> [_ w730]
                      tunnel: w724 -> [w729 w732]
                      tunnel: [w729 w731] -> w723
                      frame -1 {
                      }
                      frame Default {
                        n271 = Delete From Array(array=w732, index=w730) -> (array with subset deleted=w731:u8[])  [unwired: 1 in, 1 out]
                      }
                    }
                  }
                  frame 60..119 {
                    n272 = Search 1D Array(1D array=w740, element=w738) -> (index of element=w737:i32)  [unwired: 1 in]
                    n273 = case shown="-1" w737 {
                      tunnel: w740 -> [w741 w746]
                      tunnel: [w741 w744] -> w739
                      tunnel: w738 -> [_ w743]
                      frame 0, Default {
                      }
                      frame -1 {
                        n274 = Subtract(x=w743, y=T6 60) -> (x-y=w748:T6)
                        n275 = Insert Into Array(array=w746, new element=w743) -> (w745:u8[])  [unwired: 1 in]
                        n276 = Search 1D Array(1D array=w746, element=w748) -> (index of element=w742:i32)  [unwired: 1 in]
                        n277 = Delete From Array(array=w745, index=w742) -> (array with subset deleted=w744:u8[])  [unwired: 1 in, 1 out]
                      }
                    }
                  }
                }
              }
              n278 = call "mark_volume.vi"("element"=T6 180, "marksArray"=w691) -> ("volume"=w689:T7)  [unwired: 9 in]
              n279 = case shown="Default" w689 {
                tunnel: [w697 T2 {"type"=enum."mark", "parameter"=180.0} ("action")] -> w694
                tunnel: w693 -> [w695 _]
                tunnel: w691 -> [w696 _]
                frame Default {
                  n280 = for {
                    tunnel: [w701] -> w697
                    tunnel: w696 -> [w700]
                    tunnel: w695 -> [w698] mode=indexing
                    stop <- w699 stop-if-true
                    n281 = case shown="0..59" w698 {
                      selector: w698 -> [_ w704]
                      tunnel: [T2 {"type"=enum."empty", "parameter"=0.0} ("action") w710] -> w701
                      tunnel: w700 -> [_ w709]
                      tunnel: [FALSE TRUE] -> w699
                      frame Default {
                      }
                      frame 0..59 {
                        n282 = Add(x=w704, y=u8 120) -> (x+y=w707:u8)
                        n283 = call "mark_volume.vi"("element"=w707, "marksArray"=w709) -> ("volume"=w706:T7)  [unwired: 9 in]
                        n284 = case shown="0..1000" w706 {
                          tunnel: [T2 {"type"=enum."empty", "parameter"=0.0} ("action") w714] -> w710
                          tunnel: w707 -> [_ w713]
                          frame Default {
                          }
                          frame 0..1000 {
                            n285 = Bundle By Name(cluster=T2 {"type"=enum."mark", "parameter"=0.0} ("action"), "parameter"=w713) -> (w714:T2)
                          }
                        }
                      }
                    }
                  }
                }
                frame 0..1000 {
                }
              }
            }
          }
        }
        frame Default {
        }
      }
    }
    frame True {
      # "Ant's memory is empty"
      n286 = call "current_point_info.vi"("pieceOfWorld"=w752) -> ("marksArray"=w751:T5[])  [unwired: 2 out]
      n287 = Empty Array?(array=w751) -> (empty?=w755:bool)
      n288 = case shown="False" w755 {
        tunnel: [w763 w812] -> w756
        tunnel: [w762 w808] -> w754
        tunnel: w753 -> [_ _]
        tunnel: w751 -> [w761 _]
        frame False {
          n289 = call "mark_with_max_volume.vi"("marksArray"=w761) -> ("markValue"=w760:T5)
          n290 = Unbundle By Name(w760) -> ("volume"=w758:T7, "value"=w759:T6)
          n291 = case shown="181..194" w759 {
            selector: w759 -> [w770 w778 w786 w794 w802]
            tunnel: [w768 w782 w790 w798 w805] -> w763
            tunnel: [w774 w781 w789 w797 w803] -> w762
            tunnel: w758 -> [w769 _ _ _ _]
            frame 180 {
              w764 = T6 0 ("element")
              n292 = call "10_to_256.vi"("Decimal"=w769) -> ("256"=w773:u8[])
              n293 = Index Array(array=w773) -> (element #1=w766:u8, element #2=w767:u8, element #3=w765:u8)  [unwired: 3 in]
              n294 = Build Array(T6 180 ("element"), w766, w767, w765, w764, w764, w764) -> (w774:T6[])
              n295 = Increment(x=w770) -> (x+1=w771:T6)
              n296 = Bundle By Name(cluster=T2 {"type"=enum."mark", "parameter"=0.0} ("action"), "parameter"=w771) -> (w768:T2)
            }
            frame 181..194 {
              w776 = T6 0 ("element")
              # "Ant became a ranger"
              n297 = Increment(x=w778) -> (x+1=w780:T6)
              n298 = Subtract(x=w778, y=T6 180) -> (x-y=w777:T6)
              n299 = Build Array(w776, w777, w776, w776, w776, w776, w776, w776, w776, w776, w776, w776, w776, w776) -> (w781:T6[])
              n300 = Bundle By Name(cluster=T2 {"type"=enum."mark", "parameter"=0.0} ("action"), "parameter"=w780) -> (w782:T2)
            }
            frame 195 {
              w784 = T6 0 ("y")
              # "Ant became a ranger"
              n301 = Increment(x=w786) -> (x+1=w787:T6)
              n302 = Build Array(T6 5 ("element"), T6 0 ("element"), w784, w784, w784, w784, w784, w784, w784, w784, w784, w784, w784, w784) -> (w789:T6[])
              n303 = Bundle By Name(cluster=T2 {"type"=enum."mark", "parameter"=0.0} ("action"), "parameter"=w787) -> (w790:T2)
            }
            frame 196..240 {
              w792 = T6 0 ("element")
              # "Ant became a ranger"
              n304 = Increment(x=w794) -> (x+1=w796:T6)
              n305 = Subtract(x=w794, y=T6 181) -> (x-y=w793:T6)
              n306 = Build Array(w792, w793, w792, w792, w792, w792, w792, w792, w792, w792, w792, w792, w792, w792) -> (w797:T6[])
              n307 = Bundle By Name(cluster=T2 {"type"=enum."mark", "parameter"=0.0} ("action"), "parameter"=w796) -> (w798:T2)
            }
            frame Default {
              w800 = T6 0 ("element")
              # "Ant became an ant-on-duty"
              n308 = Build Array(T6 2 ("element"), w800, w800, w800, w800, w800, w800, w800, w800, w800, w800, w800, T6 60 ("element"), w800) -> (w803:T6[])
              n309 = Bundle By Name(cluster=T2 {"type"=enum."mark", "parameter"=0.0} ("action"), "parameter"=w802) -> (w805:T2)
            }
          }
        }
        frame True {
          w807 = T6 0 ("element")
          # "The very first ant"
          n310 = Bundle By Name(cluster=T2 {"type"=enum."mark", "parameter"=0.0} ("action"), "parameter"=T6 180 ("element")) -> (w812:T2)
          n311 = Build Array(w807, T6 0 ("element"), w807, w807, w807, w807, w807, w807, w807, w807, w807, w807, w807, w807) -> (w808:T6[])
        }
      }
    }
  }
  "error out" <- w4
  "action" <- w12
  n312 = call "memory_set.vi"("memory"=w6, "ant_base in"=w7) -> ("ant_base out"=→"Igor out":refnum<class "Igor.lvclass">)  [unwired: 8 in, 1 out]
